vi "W&R_ARDUINO2LABVIEW_nBYTES.vi"() -> ()   [LabVIEW 2019]
uses:
  <vilib>/Instr/_visa.llb/Select Event Type.ctl
  <vilib>/Instr/_visa.llb/VISA Configure Serial Port (Instr).vi
panel:
  out "error out":errorcluster
  out "read buffer":string
  in  "Numeric":i32
  out "length 2":i32
  out "length":i32
  out "concatenated string":string
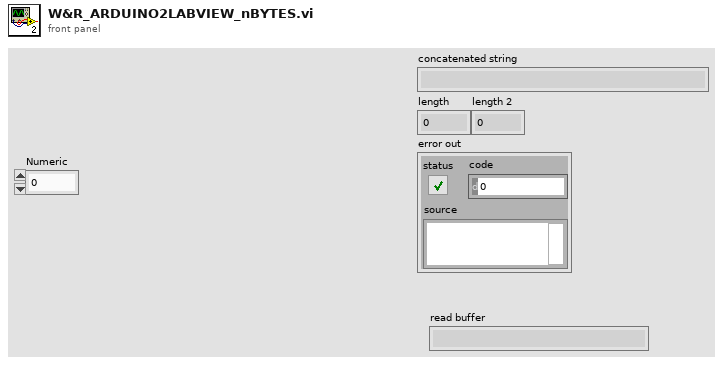
[diagram p1: front panel]
types:
  T1 = typedef "Select Event Type.ctl" = u32
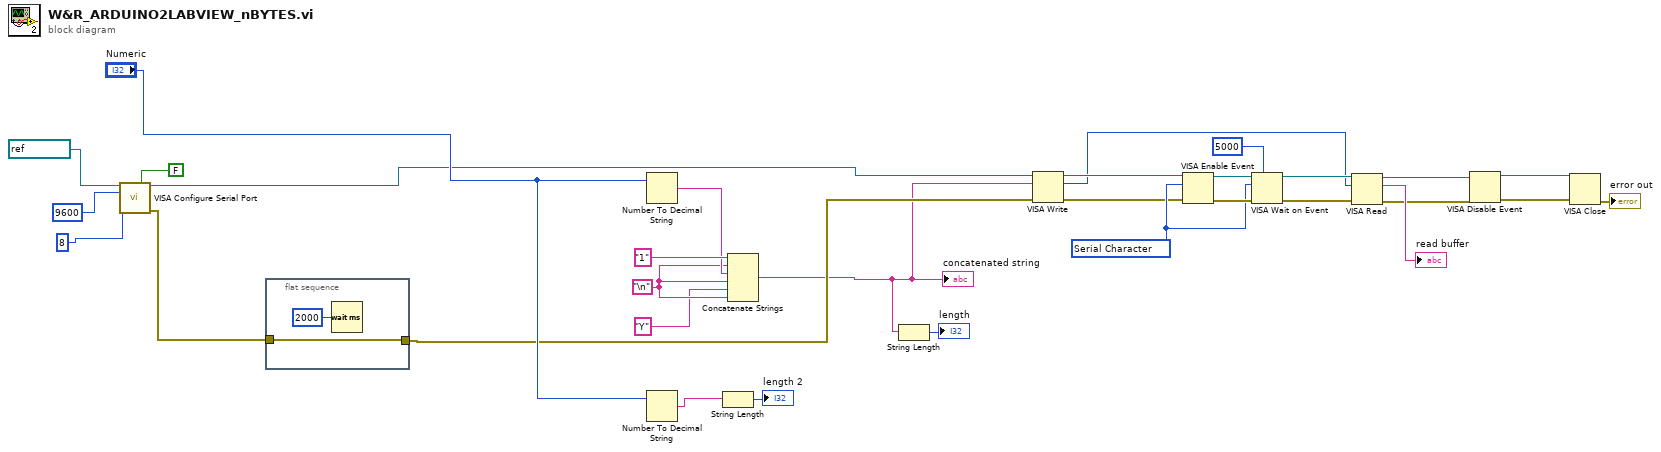
[diagram p0: block diagram]
diagram:
  w19 = T1 1073684533 items=["Service Request"=1073684491, "Trigger"=3221168138, "Clear"=1073684493, "VXI Signal"=1073684512, "VXI/VME Interrupt"=3221168161, "VXI/VME Sysfail"=1073684509, "VXI/VME Sysreset"=1073684510, "GPIB CIC"=1073684498, "GPIB Talk"=1073684499, "GPIB Listen"=1073684500, "PXI Interrupt"=1073684514, "Serial Break"=1073684515, "Serial TermChar"=1073684516, "Serial CTS"=1073684521, "Serial DSR"=1073684522, "Serial DCD"=1073684524, "Serial RI"=1073684526, "Serial Character"=1073684533, "USB Interrupt"=1073684535, "All Enabled"=1073709055] ("Event Type")
  w29 = "\n"
  n1 = call-poly "VISA Configure Serial Port"("VISA resource name"=refnum<visa-resource-name> "COM5", "Enable Termination\nChar (T)"=FALSE ("Enable Termination\nChar (T)"), "baud rate (9600)"=u32 9600, "data bits (8)"=u16 8) -> ("VISA resource name out"=w6:refnum<visa-resource-name>, "error out"=w10:errorcluster)  [unwired: 10 in]
  n2 = flat-sequence {
    tunnel: [w33] -> w8
    tunnel: w10 -> [w33]
    frame #0 {
      n3 = Wait (ms)(milliseconds to wait=u32 2000) -> ()  [unwired: 1 out]
    }
  }
  n4 = Number To Decimal String(number="Numeric") -> (decimal integer string=w30:string)  [unwired: 1 in]
  n5 = Number To Decimal String(number="Numeric") -> (decimal integer string=w26:string)  [unwired: 1 in]
  n6 = String Length(string=w26) -> (length=→"length 2":i32)
  n7 = Concatenate Strings("1", w29, w30, w29, "Y" ("string"), w29) -> (w5:string)
  "concatenated string" <- w5
  n8 = String Length(string=w5) -> (length=→"length":i32)
  n9 = VISA Write(VISA resource name=w6, write buffer=w5, error in (no error)=w8) -> (VISA resource name out=w4:refnum<visa-resource-name>, return count=w1:u32, error out=w7:errorcluster)
  n10 = VISA Enable Event(8:w7, 10:w19, 11:w4) -> (0:w23:errorcluster, 3:w22:refnum<visa-resource-name>)  [unwired: 1 in]
  n11 = VISA Wait on Event(7:u32 5000 ("timeout (0)"), 8:w23, 10:w19, 11:w22) -> (0:w20:errorcluster, 3:w21:refnum<visa-resource-name>)  [unwired: 1 in, 2 out]
  n12 = VISA Read(VISA resource name=w21, byte count=w1, error in (no error)=w20) -> (VISA resource name out=w18:refnum<visa-resource-name>, read buffer=→"read buffer":string, error out=w16:errorcluster)  [unwired: 1 out]
  n13 = VISA Disable Event(8:w16, 11:w18) -> (0:w14:errorcluster, 3:w15:refnum<visa-resource-name>)  [unwired: 2 in]
  n14 = VISA Close(VISA resource name=w15, error in (no error)=w14) -> (error out=→"error out":errorcluster)
